vi "Destroy.vi"(0 "reference in":refnum<class "Nastran PCH.lvclass">, 5 "error in (no error)":errorcluster) -> (14 "reference out":refnum<class "Nastran PCH.lvclass">, 19 "error out":errorcluster)   [LabVIEW 2022 SP3, in "Nastran PCH.lvclass"]
doc: "Destructor."
uses:
  Nastran PCH.lvclass
  API/Generic Utilities_class/Generic Utilities.lvclass
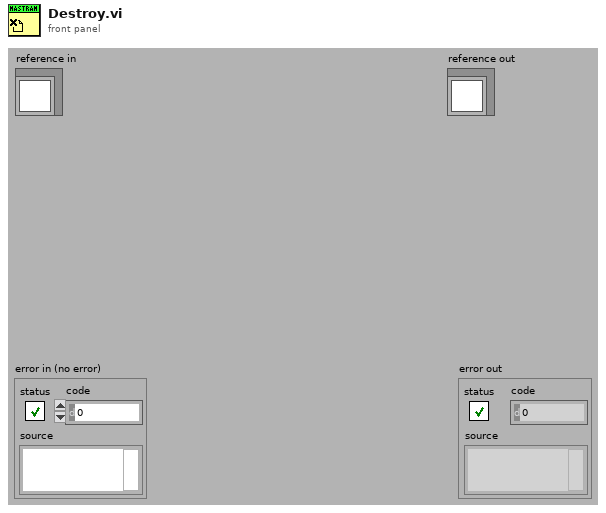
[diagram p1: front panel]
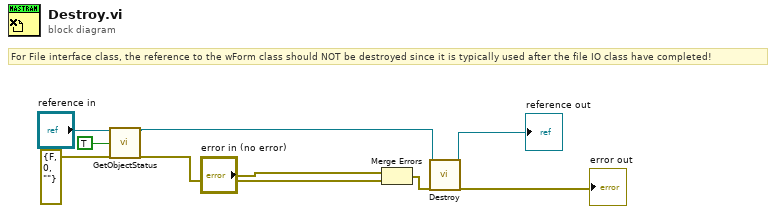
[diagram p0: block diagram]
diagram:
  # "For File interface class, the reference to the wForm class should NOT be destroyed since it is typically used after the file IO class have completed!"
  n1 = call-dynamic "GetObjectStatus.vi"("reference in"="reference in", "simple info (F)"=TRUE ("simple info"), "error in (no error)"=errorcluster {"status"=FALSE, "code"=0, "source"=""}) -> ("reference out"=w2:refnum<class "Nastran PCH.lvclass">, "error out"=w1:errorcluster)  [unwired: 5 in, 10 out]
  n2 = Merge Errors("error in (no error)", w1) -> (w8:errorcluster)
  n3 = call-parent "Destroy.vi"("reference in"=w2, "error in (no error)"=w8) -> ("reference out"=→"reference out":refnum<class "Nastran PCH.lvclass">, "error out"=→"error out":errorcluster)  [unwired: 16 in]
